vi "H5Lvisit_by_name.vi"(0 "Location Ref":T1, 1 "Index Type":T3 items=["H5_INDEX_UNKNOWN"=-1, "H5_INDEX_NAME"=0, "H5_INDEX_CRT_ORDER"=1], 2 "Order":T2 items=["H5_ITER_UNKNOWN"=-1, "H5_ITER_INC"=0, "H5_ITER_DEC"=1], 5 "Name":string=".", 7 "User data":variant, 11 "error in (no error)":errorcluster, 12 "Callback VI Ref":refnum<vi>, 13 "lapl_id":T1) -> (4 "Location Ref out":T1, 8 "User data out":variant, 15 "error out":errorcluster)   [LabVIEW 2017]
doc: "Recursively visits all links starting from a specified group."
uses:
  <vilib>/UPVI/lvhdf5/library.llb/HDF5 Ref.ctl
  <vilib>/UPVI/lvhdf5/link.llb/H5L_info_t.ctl
  <vilib>/UPVI/lvhdf5/link.llb/H5L_type_t.ctl
  <vilib>/UPVI/lvhdf5/datatype.llb/H5T_cset_t.ctl
  <vilib>/UPVI/lvhdf5/library.llb/H5_index_t.ctl
  <vilib>/UPVI/lvhdf5/library.llb/H5_iter_order_t.ctl
  <vilib>/UPVI/lvhdf5/h5helper.dll
panel:
  in  "Event Data Type":T7 {"info"."cset" items=["H5T_CSET_ERROR"=-1, "H5T_CSET_ASCII"=0, "H5T_CSET_UTF8"=1]; "info"."type" items=["H5L_TYPE_ERROR"=-1, "H5L_TYPE_HARD"=0, "H5L_TYPE_SOFT"=1, "H5L_TYPE_EXTERNAL"=64, "H5L_TYPE_MAX"=255]}
  # "LVHDF5 Toolkit\nCopyright (c) 2005-2013 by Jason D. Sommerville\nCopyright (c) 2014-2015 by UPVI, LLC.\n\nThis use and distribution of this file is governed by the terms found in \nLICENSE.txt distributed with this toolkit and installed at\n <user.lib>\\_lvhdf5\\LICENSE.txt"
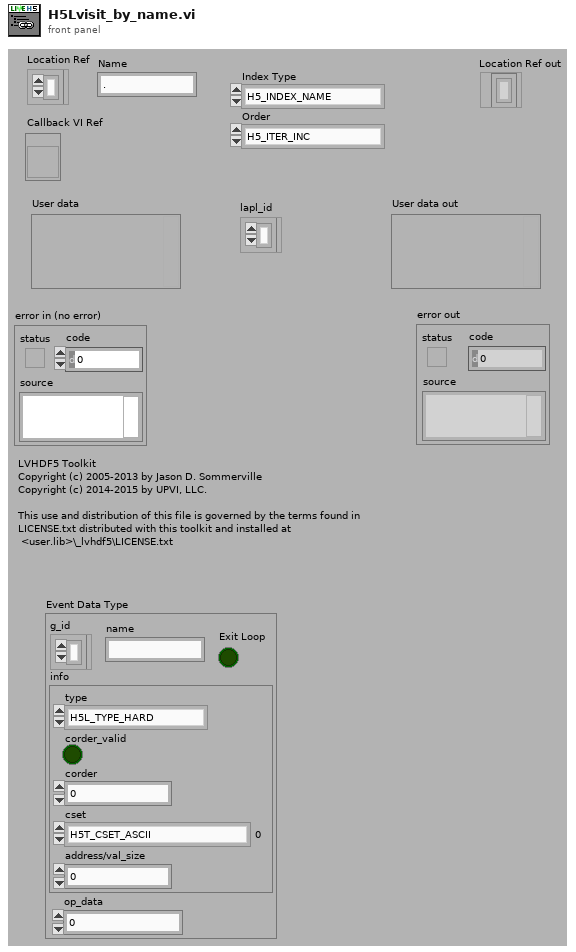
[diagram p1: front panel]
types:
  T1 = typedef "HDF5 Ref.ctl" = refnum<k1>
  T2 = typedef "H5_iter_order_t.ctl" = i32
  T3 = typedef "H5_index_t.ctl" = i32
  T4 = typedef "H5L_info_t.ctl" = cluster{"type":T5, "corder_valid":bool, "corder":i64, "cset":T6, "address/val_size":u64}
  T5 = typedef "H5L_type_t.ctl" = i32
  T6 = typedef "H5T_cset_t.ctl" = i32
  T7 = cluster{"g_id":T1, "name":string, "info":T4, "Exit Loop":bool, "op_data":u64}
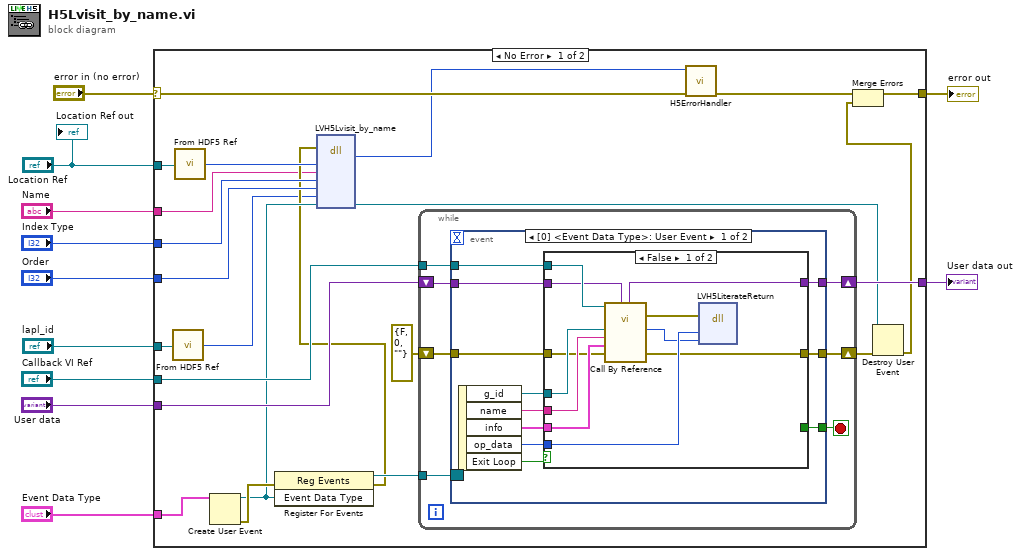
[diagram p0: block diagram]
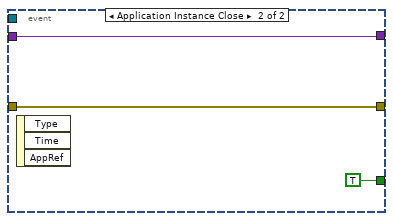
[diagram p3: hidden frame]
diagram:
  n1 = case shown="No Error" "error in (no error)" {
    selector: "error in (no error)" -> [w34 w71]
    tunnel: [w22 w71] -> w10
    tunnel: "Location Ref" -> [w32 _]
    tunnel: "Callback VI Ref" -> [w30 _]
    tunnel: "User data" -> [w29 w70]
    tunnel: "Event Data Type" -> [w26 _]
    tunnel: [w27 w70] -> w6
    tunnel: "Index Type" -> [w18 _]
    tunnel: "Order" -> [w17 _]
    tunnel: "Name" -> [w15 _]
    tunnel: "lapl_id" -> [w14 _]
    frame No Error {
      n2 = call <vilib>:"From HDF5 Ref.vi"("HDF5 Ref"=w14) -> ("I32"=w13:i32)
      n3 = call <vilib>:"From HDF5 Ref.vi"("HDF5 Ref"=w32) -> ("I32"=w24:i32)
      n4 = Create User Event(user event datatype=w26) -> (user event=w25:refnum<user-event>, error out=w31:errorcluster)  [unwired: 1 in]
      n5 = register-events(error in=w31, w25) -> (reference out=w28:refnum<event-registration>, error out=w16:errorcluster)  [unwired: 1 in]
      n6 = dll-call lib="C:/Program Files/National Instruments/LabVIEW 2017/vi.lib/UPVI/lvhdf5/h5helper.dll" fn="LVH5Lvisit_by_name" label="LVH5Literate_by_name"(error in=w16, "grp_id"=w24, "grp_name"=w15, "index_type"=w18, "order"=w17, "lapl_id"=w13, "lvevt"=w25) -> ("return type"=w33:i32, "lvevt"=w19:refnum<user-event>)  [unwired: 7 in, 2 out]
      n7 = while {
        tunnel: w28 -> [w41]
        tunnel: w30 -> [w40]
        shift-right: [w38] -> w27
        shift-left: w29 -> [w39]
        shift-right: [w36] -> w21
        shift-left: errorcluster {"status"=FALSE, "code"=0, "source"=""} ("error out") -> [w35]
        stop <- w37 stop-if-true
        n8 = event shown="[0] <Event Data Type>: User Event" {
          selector: w41 -> [_ _]
          dyn-events: _ -> [_ _]
          timeout: _ -> [_ _]
          tunnel: w40 -> [w52 _]
          tunnel: w39 -> [w48 w68]
          tunnel: [w47 w68] -> w38
          tunnel: [w46 TRUE] -> w37
          tunnel: [w43 w67] -> w36
          tunnel: w35 -> [w42 w67]
          event User Event {
            n9 = event-data() -> ("g_id"=w51:T1, "name"=w50:string, "info"=w49:T4, "op_data"=w44:u64, "Exit Loop"=w45:bool)  [unwired: 1 in]
            n10 = case shown="False" w45 {
              selector: w45 -> [_ w65]
              tunnel: w52 -> [w63 _]
              tunnel: w51 -> [w62 _]
              tunnel: w50 -> [w61 _]
              tunnel: w49 -> [w60 _]
              tunnel: w48 -> [w59 w66]
              tunnel: [w58 w66] -> w47
              tunnel: [_ w65] -> w46
              tunnel: w44 -> [w56 _]
              tunnel: [w54 w64] -> w43
              tunnel: w42 -> [w53 w64]
              frame False {
                n11 = call-by-ref "?"(reference=w63, "op_data"=w59, "error in (no error)"=w53, "info"=w60, "name"=w61, "g_id"=w62) -> (error out=w57:errorcluster, 0:"error out"=w54:errorcluster, "Stop"=w55:i32, "op_data out"=w58:variant)  [unwired: 5 in, 1 out]
                n12 = dll-call lib="C:/Program Files/National Instruments/LabVIEW 2017/vi.lib/UPVI/lvhdf5/h5helper.dll" fn="LVH5LiterateReturn"(error in=w57, "op_data"=w56, "result"=w55) -> ()  [unwired: 5 in, 2 out]
              }
              frame True {
              }
            }
          }
          event Application Instance Close {
            n13 = event-data() -> ()  [unwired: 1 in, 3 out]
          }
        }
      }
      n14 = call <vilib>:"H5ErrorHandler.vi"("error in (no error)"=w34, "herr_t"=w33) -> ("error out"=w23:errorcluster)  [unwired: 3 in, 4 out]
      n15 = Destroy User Event(user event=w19, error in=w21) -> (error out=w20:errorcluster)
      n16 = Merge Errors(w23, w20) -> (w22:errorcluster)
    }
    frame Error {
    }
  }
  "error out" <- w10
  "User data out" <- w6
  "Location Ref out" <- "Location Ref"
